vi "error.RebrandExistingError.vi"(5 "is warning? (F)":bool, 6 "maintain fatal? (T)":bool=TRUE, 7 "show call chain? (T)":bool=TRUE, 8 "error in (no error)":errorcluster, 10 "error message":string, 11 "error code (use existing)":i32) -> (0 "error out":errorcluster)   [LabVIEW 2020]
doc: "If an error occurs before this node, then it is re-branded according to the user supplied code and message.\n\nThe error details of the original error are added at the end of the new error message."
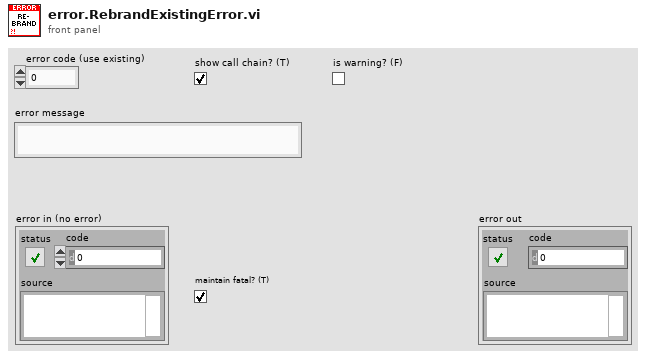
[diagram p1: front panel]
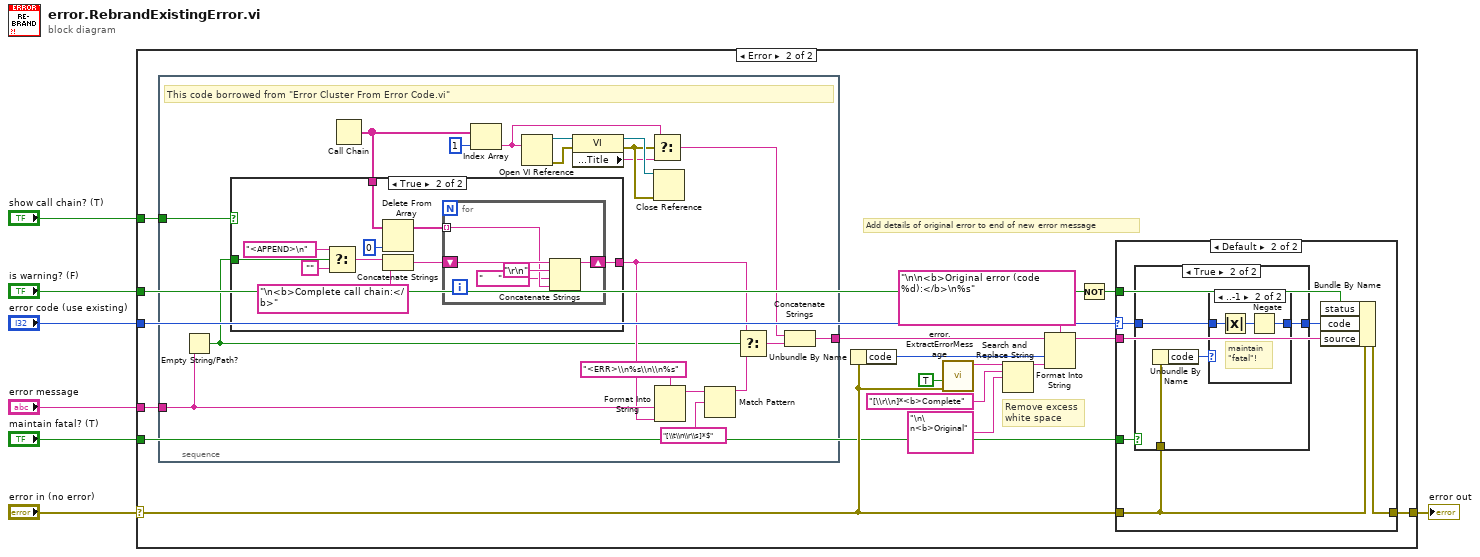
[diagram p0: block diagram]
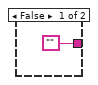
[diagram p3: hidden frame]
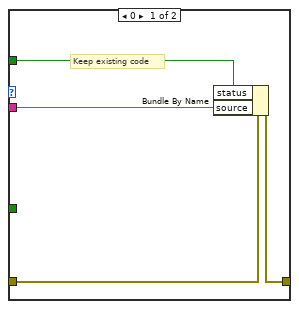
[diagram p4: hidden frame]
diagram:
  n1 = case shown="Error" "error in (no error)" {
    selector: "error in (no error)" -> [w8 w12]
    tunnel: [w8 w21] -> w2
    tunnel: "error code (use existing)" -> [_ w13]
    tunnel: "error message" -> [_ w24]
    tunnel: "show call chain? (T)" -> [_ w23]
    tunnel: "is warning? (F)" -> [_ w25]
    tunnel: "maintain fatal? (T)" -> [_ w9]
    frame No Error {
    }
    frame Error {
      # "Remove excess \nwhite space"
      # "Add details of original error to end of new error message"
      n2 = stacked-sequence {
        tunnel: w24 -> [w44]
        tunnel: w23 -> [w43]
        tunnel: [w26] -> w18
        frame #0 {
          # "This code borrowed from \"Error Cluster From Error Code.vi\""
          n3 = Empty String/Path?(string/path=w44) -> (empty?=w30:bool)
          n4 = Call Chain() -> (call chain=w38:string[])
          n5 = case shown="True" w43 {
            tunnel: ["" w55] -> w32
            tunnel: w38 -> [_ w53]
            tunnel: w30 -> [_ w49]
            frame False {
            }
            frame True {
              n6 = Select(t="<APPEND>\n", s=w49, f="") -> (s? t:f=w46:string)
              n7 = Delete From Array(array=w53, index=0) -> (array with subset deleted=w52:string[])  [unwired: 1 in, 1 out]
              n8 = Concatenate Strings(w46, "\n<b>Complete call chain:</b>" ("string")) -> (w50:string)
              n9 = for {
                tunnel: w52 -> [w57] mode=indexing
                shift-right: [w60] -> w55
                shift-left: w50 -> [w58]
                n10 = Concatenate Strings(w58, "\r\n", "     ", w57) -> (w60:string)
              }
            }
          }
          n11 = Index Array(array=w38, index=1) -> (element=w36:string)
          n12 = Open VI Reference(vi path=w36) -> (vi reference=w41:refnum<vi>, error out=w40:errorcluster)  [unwired: 5 in]
          n13 = property class="VI"(reference=w41, error in=w40) -> (reference out=w39:refnum<vi>, error out=w37:errorcluster, "Front Panel Window:Title"=w35:string)
          n14 = Select(t=w36, s=w37, f=w35) -> (s? t:f=w34:string)
          n15 = Close Reference(reference=w39, error in (no error)=w37) -> ()  [unwired: 1 out]
          n16 = Format Into String(format string="<ERR>\\n%s\\n\\n%s", w44, w32) -> (resulting string=w28:string)  [unwired: 2 in, 1 out]
          n17 = Match Pattern(string=w28, regular expression="[\\t\\n\\r\\s]*$") -> (before substring=w27:string)  [unwired: 1 in, 3 out]
          n18 = Select(t=w32, s=w30, f=w27) -> (s? t:f=w31:string)
          n19 = Concatenate Strings(w34, w31) -> (w26:string)
        }
      }
      n20 = Unbundle By Name(w12) -> ("code"=w16:i32)
      n21 = call "error.ExtractErrorMessage.vi"("error in (no error)"=w12, "include bold tags? (F)"=TRUE) -> ("error message"=w11:string)  [unwired: 9 in]
      n22 = Search and Replace String(input string=w11, search string="[\\r\\n]*<b>Complete", replace string="\n\n<b>Original" ("search string")) -> (result string=w14:string)  [unwired: 5 in, 3 out]
      n23 = Format Into String(format string="\n\n<b>Original error (code %d):</b>\n%s" ("string"), initial string=w18, w16, w14) -> (resulting string=w17:string)  [unwired: 1 in, 1 out]
      n24 = Not(x=w25) -> (.not. x?=w22:bool)
      n25 = case shown="Default" w13 {
        selector: w13 -> [_ w67]
        tunnel: w22 -> [w64 w71]
        tunnel: [w63 w70] -> w21
        tunnel: w17 -> [w62 w69]
        tunnel: w12 -> [w61 w68]
        tunnel: w9 -> [_ w65]
        frame 0 {
          # "Keep existing code"
          n26 = Bundle By Name(cluster=w61, "status"=w64, "source"=w62) -> (w63:errorcluster)
        }
        frame Default {
          n27 = case shown="True" w65 {
            tunnel: w68 -> [_ w76]
            tunnel: w67 -> [w72 w74]
            tunnel: [w72 w73] -> w66
            frame False {
            }
            frame True {
              n28 = Unbundle By Name(w76) -> ("code"=w75:i32)
              n29 = case shown="..-1" w75 {
                tunnel: w74 -> [w77 w80]
                tunnel: [w77 w78] -> w73
                frame Default {
                }
                frame ..-1 {
                  # "maintain \n\"fatal\"!"
                  n30 = Absolute Value(x=w80) -> (abs(x)=w79:i32)
                  n31 = Negate(x=w79) -> (-x=w78:i32)
                }
              }
            }
          }
          n32 = Bundle By Name(cluster=w68, "status"=w71, "code"=w66, "source"=w69) -> (w70:errorcluster)
        }
      }
    }
  }
  "error out" <- w2
